vi "Save_Time_Traces_low.vi"(0 "Use Fixed Resampling Rate":bool, 1 "Headers":T2, 2 "Put each block into separate file":bool, 3 "Precision":i16=2, 5 "method":i32(ring)=1 items=["nearest", "linear", "spline", "cubic Hermite", "Lagrange"], 7 "Data to save":i32[](array[ring]), 9 "File Extension":string=".xls", 11 "Mode":T1, 12 "Leave space between blocks?":bool, 13 "Resampling Rate Hz in":dbl=100.0, 14 "Separation Character":enum16{"Tab", "Comma"}(ring)) -> (4 "Plug in titles":string[](array[string]), 8 "Plug in values":string[](array[string]))   [LabVIEW 2022 SP3]
uses:
  Controls/File Header mode.ctl
  Controls/Average_Interpolate.ctl
  File/File Update Cluster.ctl
  <vilib>/Analysis/baseanly.llb/Mean (DBL).vi
  Globals/Meas_global.vi
  Data_plotting_vis/Results_plotter_Global.vi
  Globals/Plug_in_data_global.vi
  <vilib>/gmath/NI_Gmath.lvlib
  <vilib>/Analysis/NI_AALBase.lvlib
panel:
  out "Output:Data File:Location":string
  out "Resampling Frequency":dbl
  out "Offset:Eng:Values":dbl
  out "Scale:Eng:Values":dbl
  out "Sample:Offset:N":i32
  out "Scale:Time:":dbl
  # "These values can be provided in the Templated Results file"
  # "0 means disabled"
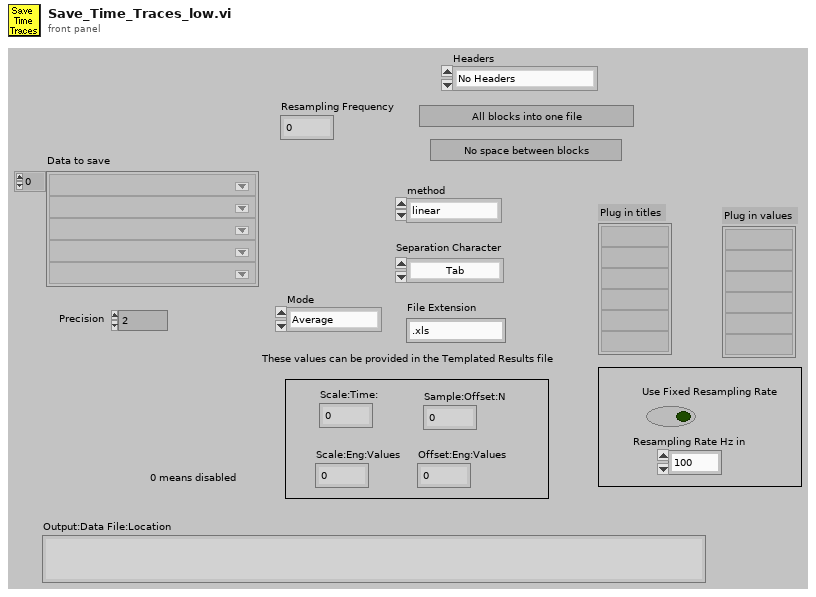
[diagram p1: front panel]
types:
  T1 = typedef "Average_Interpolate.ctl" = enum16{"Average", "Interpolate"}
  T2 = typedef "File Header mode.ctl" = enum16{"No Headers", "Headers in All files", "Separate Header File"}
  T3 = typedef "Analysis_info_cluster.ctl" = cluster{"Colour":u32, "Inst type":T4, "Inst name":string, "Symbol":string, "Code name":string, "Extra Info":string, "Inst Array":T5, "U":dbl, "u^2":dbl, "u^3":dbl, "u^4":dbl, "Skew_u":dbl, "Kurt_u":dbl, "Sd Error in Mean":dbl, "% u'/U":dbl, "X":dbl, "Y":dbl, "Z":dbl, "Timescale integral Estimate":dbl, "Sd Error in Variance":dbl, "Calib File":path, "Calib Constants":dbl[], "Output Position":bool, "Stats":enum16{"None", "Basic", "Full"}, "Av Sampling Rate":dbl, "Av No of Samples":dbl, "Total Meas Time (s)":dbl, "OrigChName":string, "Max value":dbl, "Min value":dbl, "Req Sample Rate Hz":dbl, "Sync Delay Time (s)":dbl, "Ch No":i16, "Device":string, "Use Latest Calib":bool, "Port":string, "Metadata Ch Names":string[], "Metadata Ch Values":string[], "Label":string, "chState":T6, "Point Drift":dbl, "inputConfig":string}
  T4 = typedef "Inst_type.ctl" = enum16{"Raw voltage", "Raw with zero offsetting", "Propeller anemometer", "Pressure Transducer", "Pitot-static tube", "Hot wire", "Cross wire 1", "Cross wire 2", "Generic Linear", "Generic Polynomial", "Generic BackPoly", "Fast FID", "Thermocouple", "Cold wire", "Pulsed Wire", "LDA Vel", "LDA Tran time", "LDA Arr time", "Microphone"}
  T5 = typedef "Instrument_Array.ctl" = enum16{"PWA", "LDA", "Analogue"}
  T6 = typedef "channelState.ctl" = enum32{"No Selection", "Solo", "Mute"}
  T7 = typedef "Time_Trace_Cluster.ctl" = cluster{"Weighting":dbl[], "Voltage":dbl[], "Eng Values":dbl[]}
  T8 = typedef "File Update Cluster.ctl" = cluster{"File Path":path, "Rows to Add":i32[], "Extra Ch Names":string[], "Extra Ch Values":string[], "Initial Header String":string, "Separation Character":enum16{"Tab", "Comma"}}
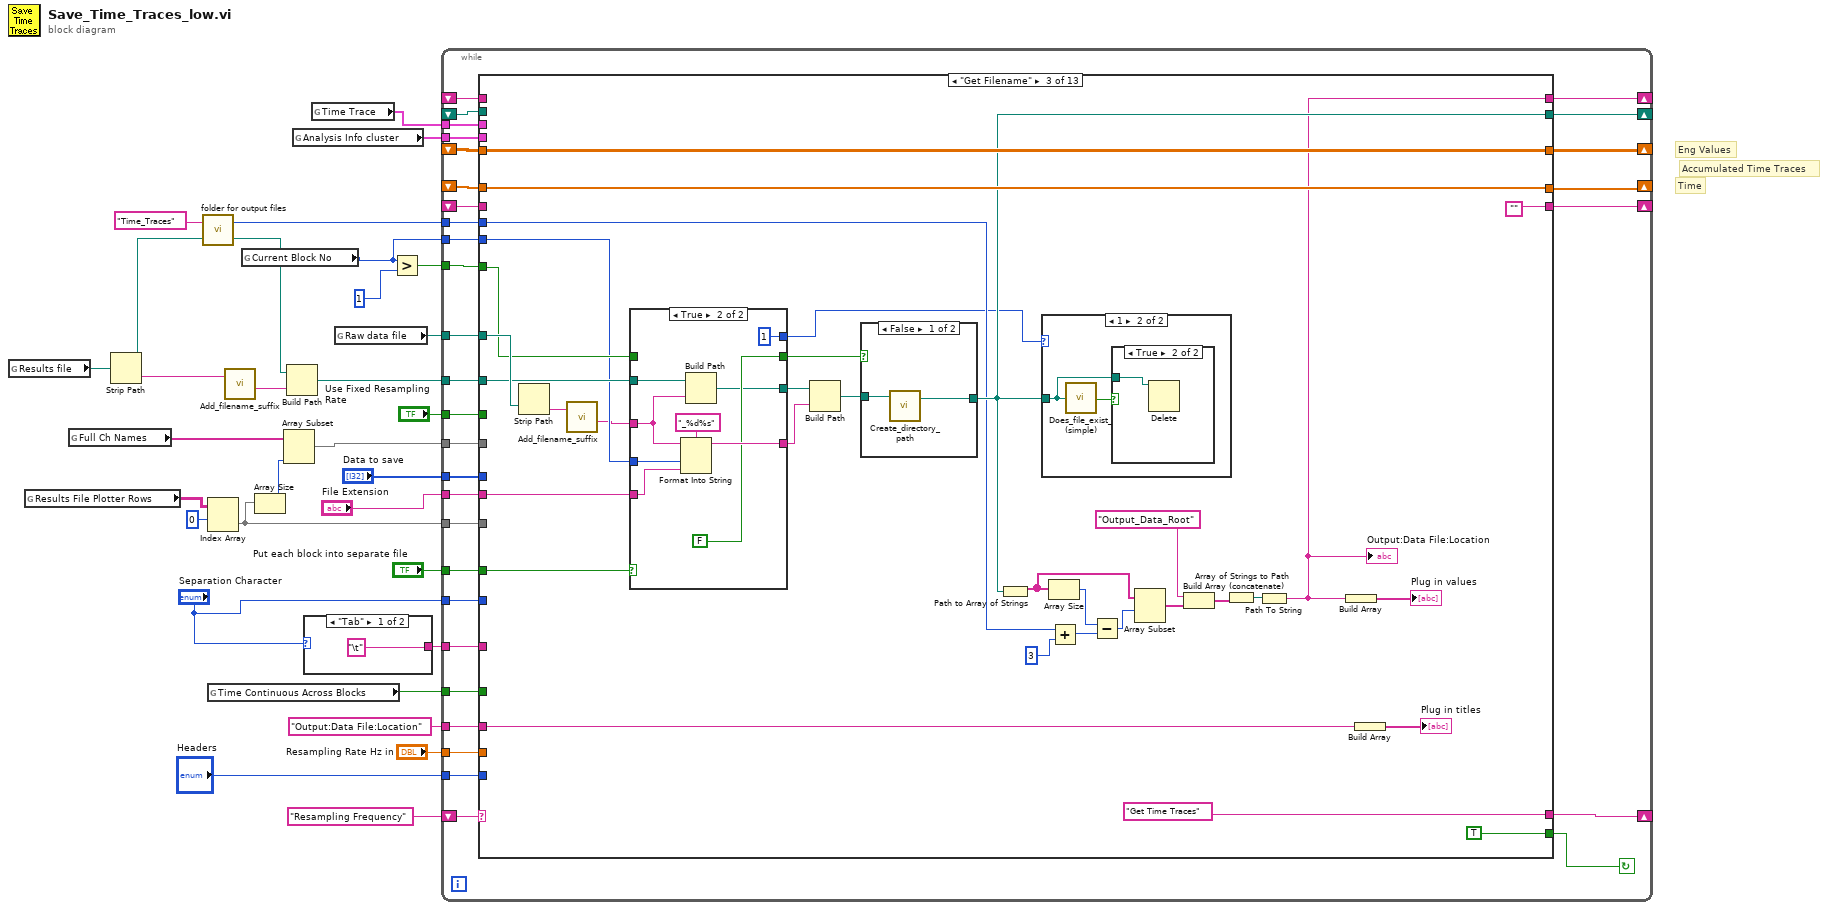
[diagram p0: block diagram]
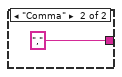
[diagram p2: hidden frame]
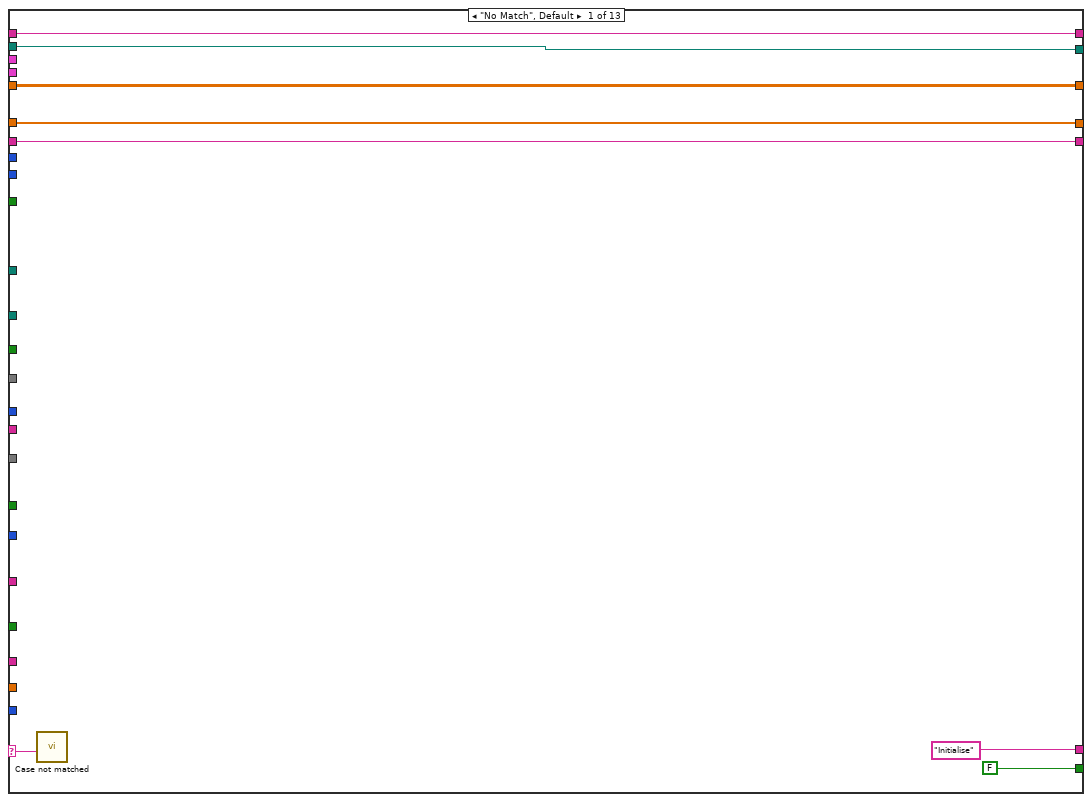
[diagram p3: hidden frame]
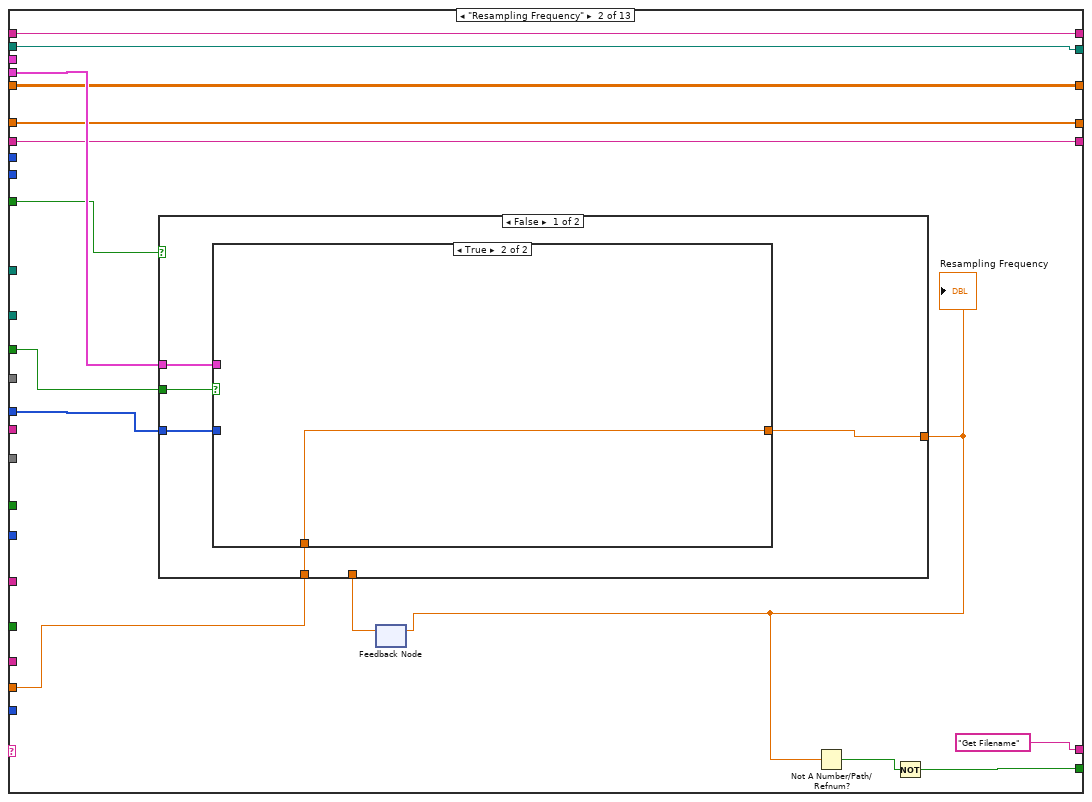
[diagram p4: hidden frame]
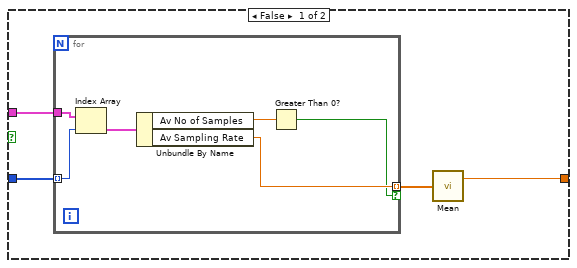
[diagram p5: hidden frame]
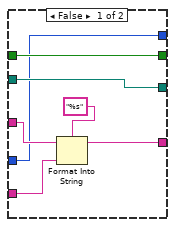
[diagram p9: hidden frame]
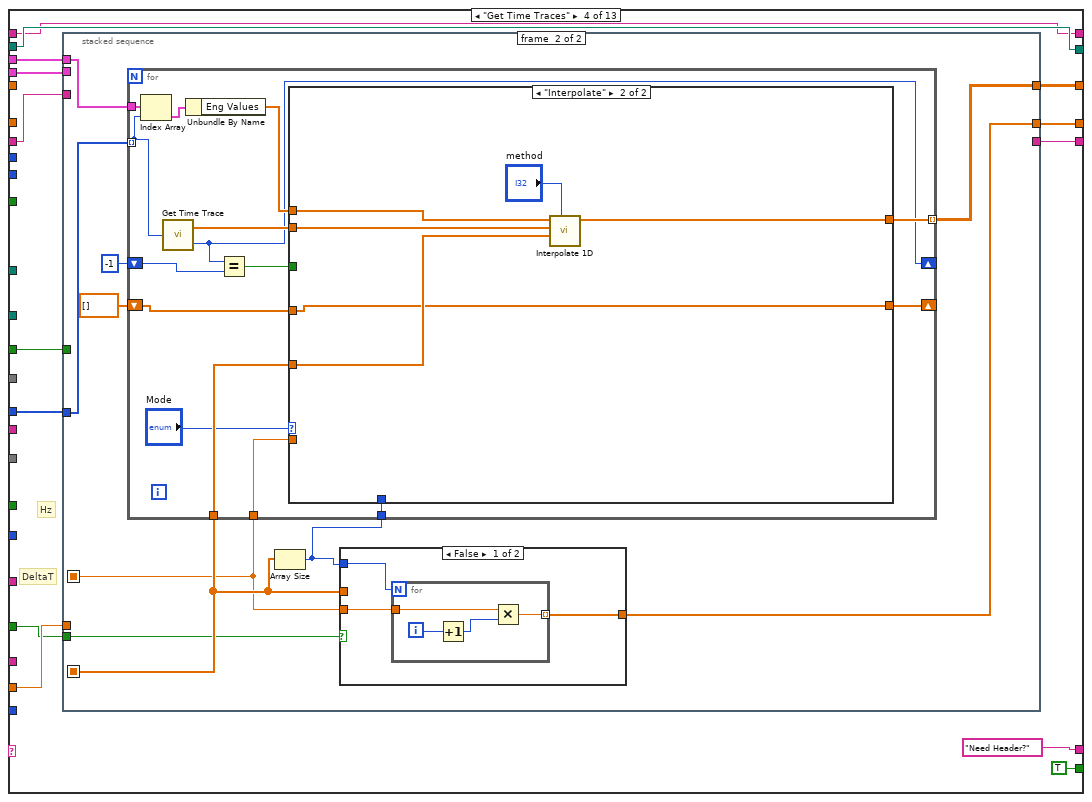
[diagram p11: hidden frame]
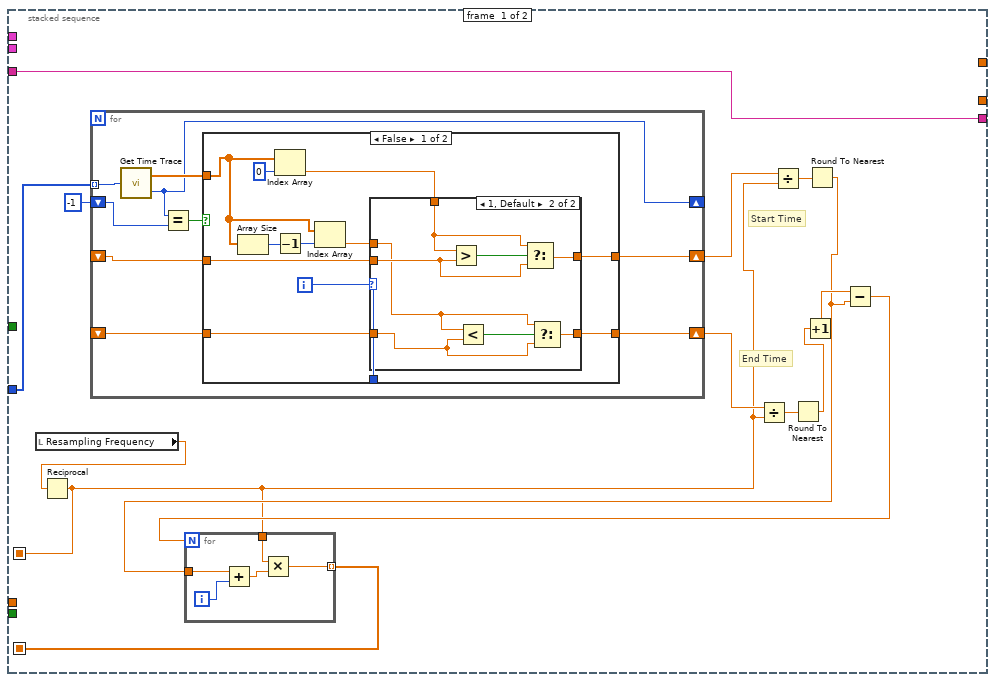
[diagram p12: hidden frame]
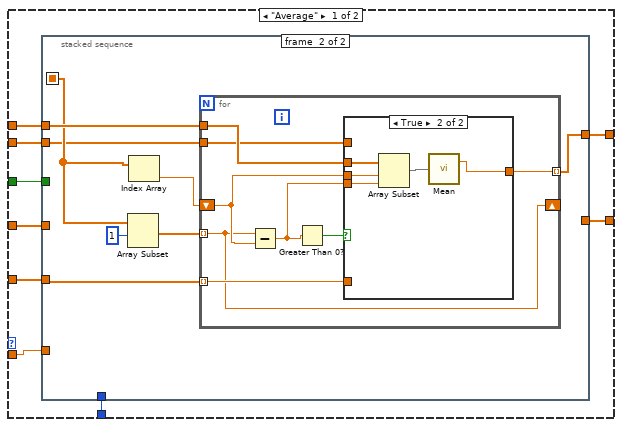
[diagram p16: hidden frame]
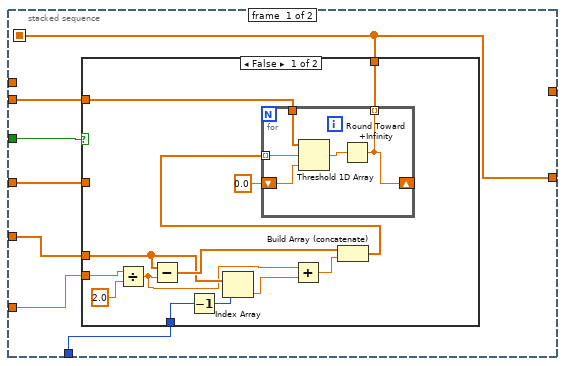
[diagram p17: hidden frame]
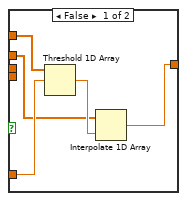
[diagram p19: hidden frame]
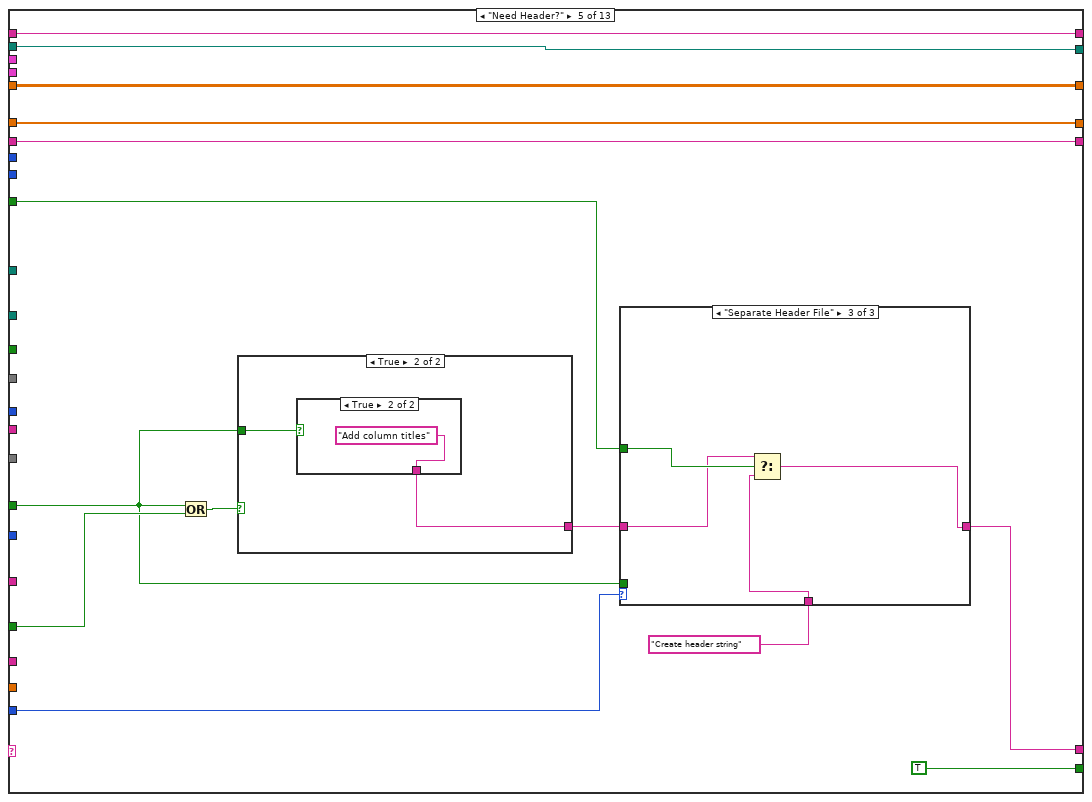
[diagram p20: hidden frame]
diagram:
  # "Accumulated Time Traces"
  # "Time"
  # "Eng Values"
  n1 = global read "Meas_global.vi" "Results file"() -> (w14:path)
  n2 = global read "Plug_in_data_global.vi" "Results File Plotter Rows"() -> (w25:string[][])
  n3 = global read "Results_plotter_Global.vi" "Full Ch Names"() -> (w21:string[])
  n4 = Strip Path(path=w14) -> (stripped path=w10:path, name=w12:string)
  n5 = call "folder for output files.vi"("results folder"=w10, "folder name"="Time_Traces" ("name or relative path")) -> ("appended path"=w5:path, "Plug_in folder depth"=w9:i32)
  n6 = Index Array(array=w25, index (row)=0) -> (element=w22:string[])  [unwired: 1 in]
  n7 = global read "Meas_global.vi" "Time Continuous Across Blocks"() -> (w17:bool)
  n8 = call "Add_filename_suffix.vi"("Filename"=w12) -> ("Base name"=w11:string)  [unwired: 1 in, 3 out]
  n9 = global read "Meas_global.vi" "Current Block No"() -> (w4:i32)
  n10 = Array Size(array=w22) -> (size(s)=w20:i32)
  n11 = Array Subset(array=w21, length=w20) -> (w19:string[])  [unwired: 1 in]
  n12 = Build Path(base path=w5, name or relative path=w11) -> (appended path=w26:path)
  n13 = global read "Meas_global.vi" "Analysis Info cluster"() -> (w18:T3[])
  n14 = case shown="\"Tab\"" "Separation Character" {
    tunnel: ["\t" ("Separation Character 2") ","] -> w16
    frame "Tab" {
    }
    frame "Comma" {
    }
  }
  n15 = global read "Meas_global.vi" "Time Trace"() -> (w3:T7[])
  n16 = global read "Meas_global.vi" "Raw data file"() -> (w27:path)
  n17 = Greater?(x=w4, y=1) -> (0:w28:bool)
  n18 = while {
    shift-left: "Resampling Frequency" -> [w38]
    shift-right: [w64] -> _
    shift-right: [w61] -> _
    shift-left: _ -> [w60]
    tunnel: "Put each block into separate file" -> [w63]
    tunnel: w27 -> [w62]
    tunnel: w28 -> [w59]
    shift-right: [w58] -> _
    shift-left: _ -> [w57]
    tunnel: w4 -> [w56]
    shift-right: [w55] -> _
    shift-left: _ -> [w54]
    tunnel: w26 -> [w53]
    tunnel: w19 -> [w52]
    tunnel: w22 -> [w51]
    tunnel: "Data to save" -> [w50]
    tunnel: w18 -> [w49]
    tunnel: w3 -> [w48]
    tunnel: w17 -> [w47]
    tunnel: w16 -> [w46]
    tunnel: "Separation Character" -> [w45]
    shift-right: [w44] -> _
    shift-left: _ -> [w43]
    shift-right: [w42] -> _
    shift-left: _ -> [w41]
    tunnel: "Output:Data File:Location" -> [w40]
    tunnel: w9 -> [w39]
    tunnel: "Use Fixed Resampling Rate" -> [w37]
    tunnel: "Resampling Rate Hz in" -> [w36]
    tunnel: "File Extension" -> [w35]
    tunnel: "Headers" -> [w34]
    stop <- w65 continue-if-true
    n19 = case shown="\"Get Filename\"" w38 {
      selector: w38 -> [w66 _ _ _ _ _ _ _ _ _ _ _ _]
      tunnel: [FALSE w77 TRUE TRUE TRUE TRUE TRUE TRUE TRUE TRUE TRUE TRUE FALSE] -> w65
      tunnel: ["Initialise" "Get Filename" "Get Time Traces" "Need Header?" w331 "Add column titles" ("t") "Sample:Offset:N" ("t") "Scale:Time:" ("t") "Scale:Eng:Values" ("t") "Offset:Eng:Values" ("t") "Create Columns" ("t") "Write File" "End" ("t")] -> w64
      tunnel: w63 -> [_ _ w134 _ w327 _ w402 _ _ _ _ _ w611]
      tunnel: w62 -> [_ _ w138 _ _ w364 _ _ _ _ _ _ _]
      tunnel: [w71 w74 "" w169 w333 w369 w417 w453 w498 w520 w542 w569 w605] -> w61
      tunnel: w60 -> [w71 w74 _ w162 w333 w369 w413 w453 w498 w520 w542 w571 w605]
      tunnel: w59 -> [_ w85 w130 _ w329 _ _ _ _ _ _ _ w609]
      tunnel: [w70 w75 w136 w171 w340 w378 w416 w452 w488 w511 w533 w564 w606] -> w58
      tunnel: w57 -> [w70 w75 w136 _ w340 w378 w416 w452 w490 w511 w533 w564 w606]
      tunnel: w56 -> [_ _ w126 _ _ _ _ _ _ _ _ _ _]
      tunnel: [w69 w76 w131 w172 w338 w377 w414 w446 w491 w512 w534 w567 w607] -> w55
      tunnel: w54 -> [w69 w76 w131 _ w338 w377 w414 w447 w491 w513 w535 w567 w607]
      tunnel: w53 -> [_ _ w128 _ _ _ _ _ _ _ _ _ _]
      tunnel: w52 -> [_ _ _ _ _ _ _ w451 w497 w519 w541 _ _]
      tunnel: w51 -> [_ _ _ _ _ _ _ w449 w495 w517 w539 _ _]
      tunnel: w50 -> [_ w87 _ w173 _ _ w410 _ _ _ _ w565 _]
      tunnel: w49 -> [_ w88 _ w174 _ _ w407 _ _ _ _ _ _]
      tunnel: w48 -> [_ _ _ w170 _ _ _ _ _ _ _ _ _]
      tunnel: w47 -> [_ _ _ w161 w335 _ _ _ _ _ _ _ w614]
      tunnel: w46 -> [_ _ _ _ _ _ w406 _ _ _ _ w559 _]
      tunnel: w45 -> [_ _ _ _ _ w371 w405 _ _ _ _ _ _]
      tunnel: [w68 w84 w118 w166 w337 w365 w404 w442 w487 w509 w531 w558 w612] -> w44
      tunnel: w43 -> [w68 w84 _ w166 w337 w365 w404 w442 w487 w509 w531 w558 w612]
      tunnel: [w67 w83 w115 w165 w336 w375 w403 w441 w486 w508 w530 w557 w608] -> w42
      tunnel: w41 -> [w67 w83 _ w165 w336 w375 w403 w441 w486 w508 w530 w557 w608]
      tunnel: w40 -> [_ _ w114 _ _ _ _ _ _ _ _ _ _]
      tunnel: w39 -> [_ _ w111 _ _ _ _ _ _ _ _ _ _]
      tunnel: w37 -> [_ w82 _ w164 _ _ _ _ _ _ _ _ _]
      tunnel: w36 -> [_ w81 _ w163 _ _ _ _ _ _ _ _ _]
      tunnel: w35 -> [_ _ w109 _ _ w363 _ _ _ _ _ _ _]
      tunnel: w34 -> [_ _ _ _ w332 w361 _ _ _ _ _ _ _]
      frame "No Match", Default {
        n20 = call "Case not matched.vi"("Case Name not Matched"=w66) -> ()
      }
      frame "Resampling Frequency" {
        n21 = feedback #1() -> (w80:dbl)  [unwired: 1 in]
        n22 = case shown="False" w85 {
          tunnel: w88 -> [w93 _]
          tunnel: w87 -> [w92 _]
          tunnel: [w91 w105] -> w79
          tunnel: w80 -> [_ w105]
          tunnel: w82 -> [w90 _]
          tunnel: w81 -> [w89 _]
          frame False {
            n23 = case shown="True" w90 {
              tunnel: w93 -> [w97 _]
              tunnel: w92 -> [w96 _]
              tunnel: [w95 w104] -> w91
              tunnel: w89 -> [_ w104]
              frame False {
                n24 = for {
                  tunnel: w97 -> [w103]
                  tunnel: [w99] -> w94 mode=indexing if=w98
                  tunnel: w96 -> [w101] mode=indexing
                  n25 = Index Array(array=w103, index=w101) -> (element=w102:T3)
                  n26 = Unbundle By Name(w102) -> ("Av No of Samples"=w100:dbl, "Av Sampling Rate"=w99:dbl)
                  n27 = Greater Than 0?(x=w100) -> (x > 0?=w98:bool)
                }
                n28 = call-poly <vilib>:"Mean.vi"("X"=w94) -> ("mean"=w95:dbl)  [unwired: 1 out]
              }
              frame True {
              }
            }
          }
          frame True {
          }
        }
        "Resampling Frequency" <- w79
        n29 = feedback-in #1(w79) -> ()
        n30 = Not A Number/Path/Refnum?(number/path/refnum=w79) -> (NaN/Path/Refnum?=w78:bool)
        n31 = Not(x=w78) -> (.not. x?=w77:bool)
      }
      frame "Get Filename" {
        n32 = Strip Path(path=w138) -> (name=w129:string)  [unwired: 1 out]
        n33 = call "Add_filename_suffix.vi"("Filename"=w129) -> ("Base name"=w110:string)  [unwired: 1 in, 3 out]
        n34 = case shown="True" w134 {
          tunnel: w110 -> [w145 w153]
          tunnel: w126 -> [w142 w151]
          tunnel: [w144 w156] -> w135
          tunnel: w130 -> [w148 _]
          tunnel: [w148 FALSE] -> w133
          tunnel: [w147 w152] -> w132
          tunnel: w128 -> [w147 w154]
          tunnel: w109 -> [w143 w150]
          tunnel: [w142 1 ("Current Block No")] -> w106
          frame False {
            n35 = Format Into String(format string="%s", initial string=w145, w143) -> (resulting string=w144:string)  [unwired: 1 in, 1 out]
          }
          frame True {
            n36 = Format Into String(format string="_%d%s", initial string=w153, w151, w150) -> (resulting string=w156:string)  [unwired: 1 in, 1 out]
            n37 = Build Path(base path=w154, name or relative path=w153) -> (appended path=w152:path)
          }
        }
        n38 = Build Path(base path=w132, name or relative path=w135) -> (appended path=w127:path)
        n39 = case shown="False" w133 {
          tunnel: w127 -> [w159 w160]
          tunnel: [w158 w160] -> w118
          frame False {
            n40 = call "Create_directory_path.vi"("Path name"=w159) -> ("Path name Out"=w158:path)  [unwired: 2 in, 1 out]
          }
          frame True {
          }
        }
        n41 = Path to Array of Strings(0:w118) -> (2:w124:string[])  [unwired: 1 out]
        n42 = case shown="1" w106 {
          tunnel: w118 -> [_ w139]
          frame Default {
          }
          frame 1 {
            n43 = call "Does_file_exist_(simple).vi"("Pathname"=w139) -> ("exists?"=w140:bool)
            n44 = case shown="True" w140 {
              tunnel: w139 -> [_ w141]
              frame False {
              }
              frame True {
                n45 = Delete(path (use dialog)=w141) -> ()  [unwired: 4 in, 3 out]
              }
            }
          }
        }
        n46 = Array Size(array=w124) -> (size(s)=w125:i32)
        n47 = Add(x=w111, y=3) -> (x+y=w112:i32)
        n48 = Subtract(x=w125, y=w112) -> (x-y=w123:i32)
        n49 = Array Subset(array=w124, index=w123) -> (w121:string[])  [unwired: 1 in]
        n50 = Build Array (concatenate)("Output_Data_Root", w121) -> (w120:string[])
        n51 = Array of Strings to Path(0:w120) -> (2:w122:path)  [unwired: 1 in]
        n52 = Path To String(path=w122) -> (string=w115:string)
        "Output:Data File:Location" <- w115
        n53 = Build Array(w115) -> (→"Plug in values":string[])
        n54 = Build Array(w114) -> (→"Plug in titles":string[])
      }
      frame "Get Time Traces" {
        # "DeltaT"
        # "Hz"
        n55 = stacked-sequence {
          seq-local: [w186 _] -> [_ w232]
          seq-local: [w179 _] -> [_ w231]
          tunnel: w174 -> [_ _]
          tunnel: w173 -> [w188 w236]
          tunnel: [_ w235] -> w172
          tunnel: [_ w233] -> w171
          tunnel: w170 -> [_ w234]
          tunnel: [w176 _] -> w169
          tunnel: w164 -> [_ _]
          tunnel: w163 -> [_ _]
          tunnel: w162 -> [w176 _]
          tunnel: w161 -> [_ w228]
          frame #0 {
            # "End Time"
            # "Start Time"
            n56 = local read "Resampling Frequency"() -> (w177:dbl)
            n57 = Reciprocal(x=w177) -> (1/x=w179:dbl)
            n58 = for {
              tunnel: w188 -> [w198] mode=indexing
              shift-right: [w201] -> w180
              shift-left: _ -> [w199]
              shift-right: [w202] -> w184
              shift-left: _ -> [w200]
              shift-right: [w196] -> _
              shift-left: -1 ("Time Array index") -> [w195]
              i -> [w203]
              n59 = call "Get Time Trace.vi"("Channel Index"=w198) -> ("Time (s)"=w197:dbl[], "Time Array index"=w196:i32)
              n60 = Equal?(x=w196, y=w195) -> (x = y?=w194:bool)
              n61 = case shown="False" w194 {
                tunnel: w203 -> [w212 _]
                tunnel: [w211 w226] -> w202
                tunnel: [w210 w225] -> w201
                tunnel: w200 -> [w206 w226]
                tunnel: w199 -> [w205 w225]
                tunnel: w197 -> [w204 _]
                frame False {
                  n62 = Array Size(array=w204) -> (size(s)=w208:i32)
                  n63 = Index Array(array=w204, index=0) -> (element=w209:dbl)
                  n64 = Decrement(x=w208) -> (x-1=w213:i32)
                  n65 = Index Array(array=w204, index=w213) -> (element=w207:dbl)
                  n66 = case shown="1, Default" w212 {
                    tunnel: [w216 w221] -> w211
                    tunnel: w209 -> [w216 w223]
                    tunnel: [w215 w217] -> w210
                    tunnel: w207 -> [w215 w219]
                    tunnel: w206 -> [_ w222]
                    tunnel: w205 -> [_ w218]
                    frame 0 {
                    }
                    frame 1, Default {
                      n67 = Greater?(x=w223, y=w222) -> (0:w224:bool)
                      n68 = Less?(x=w219, y=w218) -> (x < y?=w220:bool)
                      n69 = Select(t=w223, s=w224, f=w222) -> (s? t:f=w221:dbl)
                      n70 = Select(t=w219, s=w220, f=w218) -> (s? t:f=w217:dbl)
                    }
                  }
                }
                frame True {
                }
              }
            }
            n71 = Divide(x=w180, y=w179) -> (x/y=w181:dbl)
            n72 = Divide(x=w184, y=w179) -> (x/y=w183:dbl)
            n73 = Round To Nearest(number=w181) -> (nearest integer value=w178:dbl)
            n74 = Increment(x=w178) -> (x+1=w185:dbl)
            n75 = Round To Nearest(number=w183) -> (nearest integer value=w182:dbl)
            n76 = Subtract(x=w185, y=w182) -> (x-y=w187:dbl)
            n77 = for {
              N: w187 -> [_]
              tunnel: w182 -> [w192]
              tunnel: w179 -> [w190]
              tunnel: [w189] -> w186 mode=indexing
              i -> [w193]
              n78 = Add(x=w192, y=w193) -> (x+y=w191:dbl)
              n79 = Multiply(x=w190, y=w191) -> (x*y=w189:dbl)
            }
          }
          frame #1 {
            n80 = Array Size(array=w232) -> (size(s)=w227:i32)
            n81 = for {
              tunnel: w234 -> [w259]
              tunnel: w236 -> [w254] mode=indexing
              tunnel: w232 -> [w256]
              tunnel: [w255] -> w235 mode=indexing
              tunnel: w231 -> [w252]
              tunnel: w227 -> [w251]
              shift-right: [w250] -> _
              shift-left: -1 ("Time Array index") -> [w249]
              shift-right: [w247] -> _
              shift-left: dbl[] [] -> [w246]
              n82 = Index Array(array=w259, index=w254) -> (element=w258:T7)
              n83 = call "Get Time Trace.vi"("Channel Index"=w254) -> ("Time (s)"=w253:dbl[], "Time Array index"=w250:i32)
              n84 = Unbundle By Name(w258) -> ("Eng Values"=w257:dbl[])
              n85 = Equal?(x=w250, y=w249) -> (x = y?=w248:bool)
              n86 = case shown="\"Interpolate\"" "Mode" {
                tunnel: w257 -> [w264 w326]
                tunnel: w256 -> [w266 w325]
                tunnel: [w263 w323] -> w255
                tunnel: w253 -> [w268 w322]
                tunnel: w252 -> [w267 _]
                tunnel: w251 -> [w265 _]
                tunnel: w248 -> [w262 _]
                tunnel: [w261 w321] -> w247
                tunnel: w246 -> [w260 w321]
                frame "Average" {
                  n87 = stacked-sequence {
                    seq-local: [w270 _] -> [_ w300]
                    tunnel: w268 -> [w275 w296]
                    tunnel: w267 -> [w274 _]
                    tunnel: w266 -> [w273 w297]
                    tunnel: w265 -> [w272 _]
                    tunnel: w264 -> [_ w302]
                    tunnel: [_ w295] -> w263
                    tunnel: w262 -> [w271 _]
                    tunnel: [w270 _] -> w261
                    tunnel: w260 -> [w269 _]
                    frame #0 {
                      n88 = case shown="False" w271 {
                        tunnel: w275 -> [w288 _]
                        tunnel: w274 -> [w285 _]
                        tunnel: w273 -> [w283 _]
                        tunnel: w272 -> [w277 _]
                        tunnel: [w278 w294] -> w270
                        tunnel: w269 -> [_ w294]
                        frame False {
                          n89 = Divide(x=w285, y=2.0) -> (x/y=w281:dbl)
                          n90 = Subtract(x=w283, y=w281) -> (x-y=w284:dbl[])
                          n91 = Decrement(x=w277) -> (x-1=w276:i32)
                          n92 = Index Array(array=w283, index=w276) -> (element=w282:dbl)
                          n93 = Add(x=w281, y=w282) -> (x+y=w280:dbl)
                          n94 = Build Array (concatenate)(w284, w280) -> (w279:dbl[])
                          n95 = for {
                            tunnel: w288 -> [w293]
                            tunnel: w279 -> [w292] mode=indexing
                            shift-right: [w289] -> _
                            shift-left: 0.0 -> [w290]
                            tunnel: [w289] -> w278 mode=indexing
                            n96 = Threshold 1D Array(1:w290, 2:w292, 3:w293) -> (0:w291:dbl)
                            n97 = Round Toward +Infinity(x=w291) -> (ceil(x): smallest int >= x=w289:dbl)
                          }
                        }
                        frame True {
                        }
                      }
                    }
                    frame #1 {
                      n98 = Array Subset(array=w300, index=1) -> (w298:dbl[])  [unwired: 1 in]
                      n99 = Index Array(array=w300) -> (element=w299:dbl)  [unwired: 1 in]
                      n100 = for {
                        tunnel: w302 -> [w310]
                        tunnel: [w309] -> w295 mode=indexing
                        shift-right: [w303] -> _
                        shift-left: w299 -> [w304]
                        tunnel: w298 -> [w303] mode=indexing
                        tunnel: w297 -> [w306] mode=indexing
                        tunnel: w296 -> [w305]
                        n101 = Subtract(x=w303, y=w304) -> (x-y=w308:dbl)
                        n102 = Greater Than 0?(x=w308) -> (x > 0?=w307:bool)
                        n103 = case shown="True" w307 {
                          tunnel: w310 -> [w312 w320]
                          tunnel: [w311 w318] -> w309
                          tunnel: w304 -> [_ w317]
                          tunnel: w308 -> [_ w316]
                          tunnel: w306 -> [w314 _]
                          tunnel: w305 -> [w315 _]
                          frame False {
                            n104 = Threshold 1D Array(2:w314, 3:w315) -> (0:w313:dbl)  [unwired: 1 in]
                            n105 = Interpolate 1D Array(1:w313, 2:w312) -> (0:w311:dbl)
                          }
                          frame True {
                            n106 = Array Subset(array=w320, index=w317, length=w316) -> (w319:dbl[])
                            n107 = call-poly <vilib>:"Mean.vi"("X"=w319) -> ("mean"=w318:dbl)  [unwired: 1 out]
                          }
                        }
                      }
                    }
                  }
                }
                frame "Interpolate" {
                  n108 = call <vilib>:"Interpolate 1D.vi"("method"="method", "xi"=w325, "X"=w322, "Y"=w326) -> ("yi"=w323:dbl[])  [unwired: 2 in, 5 out]
                }
              }
            }
            n109 = case shown="False" w228 {
              tunnel: [w239 w244] -> w233
              tunnel: w232 -> [_ w244]
              tunnel: w231 -> [w238 _]
              tunnel: w227 -> [w237 _]
              frame False {
                n110 = for {
                  N: w237 -> [_]
                  tunnel: w238 -> [w243]
                  tunnel: [w242] -> w239 mode=indexing
                  i -> [w241]
                  n111 = Increment(x=w241) -> (x+1=w240:i32)
                  n112 = Multiply(x=w243, y=w240) -> (x*y=w242:dbl)
                }
              }
              frame True {
              }
            }
          }
        }
      }
      frame "Need Header?" {
        n113 = Or(x=w327, y=w335) -> (x .or. y?=w334:bool)
        n114 = case shown="True" w334 {
          tunnel: ["Sample:Offset:N" ("t") w357] -> w330
          tunnel: w327 -> [_ w358]
          frame False {
          }
          frame True {
            n115 = case shown="True" w358 {
              tunnel: ["Sample:Offset:N" ("t") "Add column titles" ("t")] -> w357
              frame False {
              }
              frame True {
              }
            }
          }
        }
        n116 = case shown="\"Separate Header File\"" w332 {
          tunnel: [w341 w345 w352] -> w331
          tunnel: w330 -> [w341 w342 w354]
          tunnel: w329 -> [_ w343 w355]
          tunnel: "Create header string" -> [_ w344 w353]
          tunnel: w327 -> [_ w346 _]
          frame "No Headers" {
          }
          frame "Headers in All files" {
            n117 = case shown="True" w346 {
              tunnel: [w347 w351] -> w345
              tunnel: w344 -> [w348 w351]
              tunnel: w343 -> [w350 _]
              tunnel: w342 -> [w349 _]
              frame False {
                n118 = Select(t=w349, s=w350, f=w348) -> (s? t:f=w347:string)
              }
              frame True {
              }
            }
          }
          frame "Separate Header File" {
            n119 = Select(t=w354, s=w355, f=w353) -> (s? t:f=w352:string)
          }
        }
      }
      frame "Create header string" {
        w374 = string[] [] ("Extra Ch Names")
        n120 = case shown="\"Separate Header File\"" w361 {
          tunnel: w365 -> [w383 w394]
          tunnel: w364 -> [_ w391]
          tunnel: w363 -> [_ w388]
          tunnel: [w383 w384] -> w362
          frame Default {
          }
          frame "Separate Header File" {
            n121 = Strip Path(path=w391) -> (name=w392:string)  [unwired: 1 out]
            n122 = call "Add_filename_suffix.vi"("Filename"=w392) -> ("Base name"=w390:string)  [unwired: 1 in, 3 out]
            n123 = Strip Path(path=w394) -> (stripped path=w393:path)  [unwired: 1 out]
            n124 = Concatenate Strings(w390, "_header" ("string"), w388) -> (w387:string)
            n125 = Build Path(base path=w393, name or relative path=w387) -> (appended path=w385:path)
            n126 = call "Does_file_exist_(simple).vi"("Pathname"=w385) -> ("exists?"=w386:bool)
            n127 = case shown="False" w386 {
              tunnel: w385 -> [w395 w397]
              tunnel: [w395 w396] -> w384
              frame False {
              }
              frame True {
                n128 = Delete(path (use dialog)=w397) -> (deleted path=w396:path)  [unwired: 4 in, 2 out]
              }
            }
          }
        }
        n129 = global read "Meas_global.vi" "Duplicate channels"() -> (w368:i32[])
        n130 = Array Size(array=w368) -> (size(s)=w367:i32)
        n131 = case shown="0" w367 {
          selector: w367 -> [_ w400]
          tunnel: [i32[] [0] ("Rows to Add") w399] -> w366
          frame 0 {
          }
          frame Default {
            n132 = for {
              N: w400 -> [_]
              tunnel: [w401] -> w399 mode=indexing
              i -> [w401]
            }
          }
        }
        n133 = Bundle By Name(cluster=T8 {"File Path"=path "", "Rows to Add"=[], "Extra Ch Names"=[], "Extra Ch Values"=[], "Initial Header String"="", "Separation Character"=enum."Tab"} ("File to Update"), "Initial Header String"="", "File Path"=w362, "Extra Ch Names"=w374, "Extra Ch Values"=w374, "Separation Character"=w371, "Rows to Add"=w366) -> (w370:T8)
        n134 = case shown="Default" w361 {
          tunnel: w370 -> [_ w381]
          frame "No Headers" {
          }
          frame Default {
            n135 = global read "Meas_global.vi" "Files to Update"() -> (w382:T8[])
            n136 = Build Array (concatenate)(w382, w381) -> (w380:T8[])
            n137 = global write "Meas_global.vi" "Files to Update"(w380) -> ()
          }
        }
      }
      frame "Add column titles" {
        n138 = for {
          tunnel: [w440] -> w412 mode=indexing
          tunnel: w410 -> [w439] mode=indexing
          tunnel: w407 -> [w438]
          n139 = Index Array(array=w438, index=w439) -> (element=w437:T3)
          n140 = Unbundle By Name(w437) -> ("Inst name"=w440:string)
        }
        n141 = Build Array (concatenate)("Time (s)", w412) -> (w411:string[])
        n142 = Array To Spreadsheet String(delimiter (Tab)=w406, array=w411, 3:"%s" ("format string")) -> (spreadsheet string=w415:string)
        n143 = case shown="\"Comma\"" w405 {
          tunnel: [w425 w436] -> w417
          tunnel: w415 -> [w424 w435]
          tunnel: w413 -> [w423 w431]
          tunnel: w402 -> [w422 _]
          frame "Comma" {
            n144 = case shown="True" w422 {
              tunnel: [w426 ""] -> w421
              tunnel: [w426 "\r\n"] -> w420
              frame False {
                w426 = "\r\n"
              }
              frame True {
              }
            }
            n145 = Concatenate Strings(w423, w421, w424, w420) -> (w425:string)
          }
          frame "Tab" {
            w429 = "\r\n"
            n146 = Initialize Array("", 10) -> (w432:string[])
            n147 = call "Asterisk_header.vi"("Channel names"=w432) -> ("Header string"=w430:string)
            n148 = Concatenate Strings(w431, w429, w430, w429, w429, w435, w429, w429) -> (w436:string)
          }
        }
      }
      frame "Sample:Offset:N" {
        n149 = Search 1D Array(1D array=w451, element="Sample:Offset:N") -> (index of element=w448:i32)  [unwired: 1 in]
        n150 = case shown="Default" w448 {
          tunnel: w449 -> [w461 _]
          tunnel: w448 -> [w460 _]
          tunnel: w447 -> [w458 w485]
          tunnel: [w456 w485] -> w446
          tunnel: [w454 0] -> w443
          frame Default {
            n151 = Index Array(array=w461, index=w460) -> (element=w459:string)
            n152 = Fract/Exp String To Number(string=w459, default (0 dbl)=0 ("default (0 DBL)")) -> (number=w454:i32)  [unwired: 2 in, 1 out]
            n153 = Greater Than 0?(x=w454) -> (x > 0?=w455:bool)
            n154 = case shown="False" w455 {
              tunnel: w458 -> [w464 w475]
              tunnel: w454 -> [w463 w474]
              tunnel: [w462 w473] -> w456
              frame True {
                n155 = for {
                  tunnel: w464 -> [w468] mode=indexing
                  tunnel: w463 -> [w470]
                  tunnel: [w465] -> w462 mode=indexing
                  n156 = Array Size(array=w468) -> (size(s)=w471:i32)
                  n157 = Array Subset(array=w468, length=w470) -> (w472:dbl[])  [unwired: 1 in]
                  n158 = Reverse 1D Array(array=w472) -> (reversed array=w467:dbl[])
                  n159 = Subtract(x=w471, y=w470) -> (x-y=w469:i32)
                  n160 = Array Subset(array=w468, length=w469) -> (w466:dbl[])  [unwired: 1 in]
                  n161 = Build Array (concatenate)(w467, w466) -> (w465:dbl[])
                }
              }
              frame False {
                n162 = for {
                  tunnel: w475 -> [w482] mode=indexing
                  tunnel: w474 -> [w480]
                  tunnel: [w481] -> w473 mode=indexing
                  n163 = Array Size(array=w482) -> (size(s)=w483:i32)
                  n164 = Array Subset(array=w482, index=w480) -> (w479:dbl[])  [unwired: 1 in]
                  n165 = Subtract(x=w483, y=w480) -> (x-y=w478:i32)
                  n166 = Array Subset(array=w482, index=w478) -> (w477:dbl[])  [unwired: 1 in]
                  n167 = Reverse 1D Array(array=w477) -> (reversed array=w476:dbl[])
                  n168 = Build Array (concatenate)(w479, w476) -> (w481:dbl[])
                }
              }
            }
          }
          frame -1 {
          }
        }
        "Sample:Offset:N" <- w443
      }
      frame "Scale:Time:" {
        n169 = Search 1D Array(1D array=w497, element="Scale:Time:") -> (index of element=w494:i32)  [unwired: 1 in]
        n170 = case shown="Default" w494 {
          tunnel: w495 -> [w505 _]
          tunnel: w494 -> [w504 _]
          tunnel: w490 -> [w501 w507]
          tunnel: [w500 w507] -> w488
          tunnel: [w499 1.0] -> w489
          frame Default {
            n171 = Index Array(array=w505, index=w504) -> (element=w503:string)
            n172 = Fract/Exp String To Number(string=w503, default (0 dbl)=0.0 ("default (0 DBL)")) -> (number=w499:dbl)  [unwired: 2 in, 1 out]
            n173 = Multiply(x=w501, y=w499) -> (x*y=w500:dbl[])
          }
          frame -1 {
          }
        }
        "Scale:Time:" <- w489
      }
      frame "Scale:Eng:Values" {
        n174 = Search 1D Array(1D array=w519, element="Scale:Eng:Values") -> (index of element=w516:i32)  [unwired: 1 in]
        n175 = case shown="-1" w516 {
          tunnel: w517 -> [w527 _]
          tunnel: w516 -> [w526 _]
          tunnel: w513 -> [w523 w529]
          tunnel: [w522 w529] -> w512
          tunnel: [w521 1.0] -> w510
          frame Default {
            n176 = Index Array(array=w527, index=w526) -> (element=w525:string)
            n177 = Fract/Exp String To Number(string=w525, default (0 dbl)=0.0 ("default (0 DBL)")) -> (number=w521:dbl)  [unwired: 2 in, 1 out]
            n178 = Multiply(x=w523, y=w521) -> (x*y=w522:dbl[][])
          }
          frame -1 {
          }
        }
        "Scale:Eng:Values" <- w510
      }
      frame "Offset:Eng:Values" {
        n179 = Search 1D Array(1D array=w541, element="Offset:Eng:Values") -> (index of element=w538:i32)  [unwired: 1 in]
        n180 = case shown="Default" w538 {
          tunnel: w539 -> [w549 _]
          tunnel: w538 -> [w548 _]
          tunnel: w535 -> [w545 w551]
          tunnel: [w544 w551] -> w534
          tunnel: [w543 0.0] -> w532
          frame Default {
            n181 = Index Array(array=w549, index=w548) -> (element=w547:string)
            n182 = Fract/Exp String To Number(string=w547, default (0 dbl)=0.0 ("default (0 DBL)")) -> (number=w543:dbl)  [unwired: 2 in, 1 out]
            n183 = Add(x=w545, y=w543) -> (x+y=w544:dbl[][])
          }
          frame -1 {
          }
        }
        "Offset:Eng:Values" <- w532
      }
      frame "Create Columns" {
        n184 = Index Array(array=w564, index #1=1 ("index"), index #2=0 ("index")) -> (element #1=w563:dbl, element #2=w562:dbl)
        n185 = Array Size(array=w565) -> (size(s)=w573:i32)
        n186 = Subtract(x=w563, y=w562) -> (x-y=w556:dbl)
        n187 = Reciprocal(x=w556) -> (1/x=w555:dbl)
        n188 = Number To Decimal String(number=w555) -> (decimal integer string=w554:string)  [unwired: 1 in]
        n189 = String Length(string=w554) -> (length=w553:i32)
        n190 = Increment(x=w553) -> (x+1=w552:i32)
        n191 = Decrement(x=w573) -> (x-1=w574:i32)
        n192 = for {
          shift-right: [w588] -> w570
          shift-left: "" -> [w583]
          tunnel: w559 -> [w576]
          tunnel: w567 -> [w586]
          tunnel: w574 -> [w582]
          tunnel: w564 -> [w579] mode=indexing
          tunnel: w552 -> [w578]
          i -> [w580]
          n193 = Index Array(array=w586, index (col)=w580) -> (element=w585:dbl[])  [unwired: 1 in]
          n194 = Number To Fractional String(number=w579, precision (6)=w578) -> (F-format string=w577:string)  [unwired: 2 in]
          n195 = Concatenate Strings(w577, w576) -> (w575:string)
          n196 = for {
            shift-right: [w595] -> w584
            shift-left: w575 -> [w597]
            tunnel: w576 -> [w594]
            tunnel: w585 -> [w589] mode=indexing
            tunnel: w582 -> [w593]
            tunnel: "Precision" -> [w591]
            i -> [w590]
            n197 = Equal?(x=w590, y=w593) -> (x = y?=w592:bool)
            n198 = Number To Fractional String(number=w589, precision (6)=w591) -> (F-format string=w596:string)  [unwired: 2 out]
            n199 = case shown="False" w592 {
              tunnel: w597 -> [w601 w604]
              tunnel: w596 -> [w600 w603]
              tunnel: [w599 w602] -> w595
              tunnel: w594 -> [w598 _]
              frame False {
                n200 = Concatenate Strings(w601, w600, w598) -> (w599:string)
              }
              frame True {
                n201 = Concatenate Strings(w604, w603) -> (w602:string)
              }
            }
          }
          n202 = Concatenate Strings(w583, w584, "\r\n") -> (w588:string)
        }
        n203 = Concatenate Strings(w571, w570) -> (w569:string)
      }
      frame "Write File" {
        n204 = case shown="False" w614 {
          tunnel: ["Leave space between blocks?" FALSE] -> w613
          frame False {
          }
          frame True {
          }
        }
        n205 = case shown="False" w611 {
          tunnel: [w621 FALSE] -> w610
          tunnel: w609 -> [w621 _]
          frame False {
          }
          frame True {
          }
        }
        n206 = case shown="True" w610 {
          tunnel: [w625 w630] -> w619
          tunnel: w605 -> [w625 w629]
          tunnel: [w626 w628] -> w620
          tunnel: w613 -> [_ w627]
          frame False {
            w626 = FALSE  # append to file? (new file:F)
          }
          frame True {
            w628 = TRUE  # append to file? (new file:F)
            n207 = case shown="True" w627 {
              tunnel: [w631 w634] -> w630
              tunnel: w629 -> [w631 w633]
              frame False {
              }
              frame True {
                n208 = Concatenate Strings("\r\n", w633) -> (w634:string)
              }
            }
          }
        }
        n209 = global read "Meas_global.vi" "Iteration Number"() -> (w616:i32)
        n210 = Equal To 0?(x=w616) -> (x = 0?=w615:bool)
        n211 = call "Write_Characters_To_File.vi"("file path (dialog if empty)"=w612, "advisory dialog? (display:T)"=w615, "character string"=w619, "append to file? (new file:F)"=w620) -> ()  [unwired: 1 in, 4 out]
      }
    }
  }
